vi "Write Time Measurement Requested 2.vi"(8 "error in (no error)":errorcluster, 10 "Time Measurement Requested":timestamp, 11 "Launch Measurements Message in":refnum<class "Launch Measurements Message.lvclass">) -> (0 "error out":errorcluster, 3 "Launch Measurements Message out":refnum<class "Launch Measurements Message.lvclass">)   [LabVIEW 2015, in "Controller Actor.lvlib" / "Launch Measurements Message.lvclass"]
uses:
  Launch Measurements Message.lvclass
  Launch Measurements Message.lvclass/Launch Measurements Message.ctl
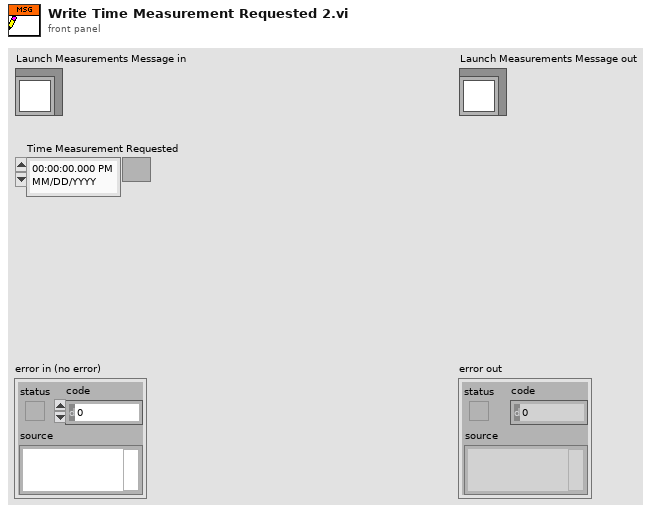
[diagram p1: front panel]
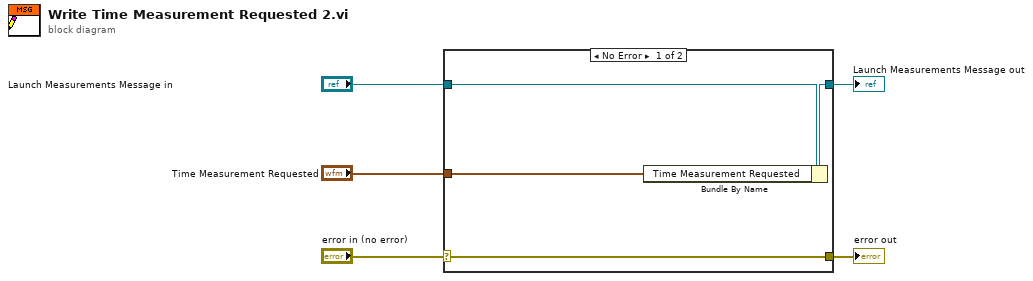
[diagram p0: block diagram]
diagram:
  n1 = case shown="No Error" "error in (no error)" {
    selector: "error in (no error)" -> [w9 w10]
    tunnel: [w9 w10] -> w4
    tunnel: [w7 w11] -> w2
    tunnel: "Launch Measurements Message in" -> [w8 w11]
    tunnel: "Time Measurement Requested" -> [w6 _]
    frame No Error {
      n2 = Bundle By Name(cluster=w8, "Time Measurement Requested"=w6) -> (w7:refnum<class "Launch Measurements Message.lvclass">)
    }
    frame Error {
    }
  }
  "error out" <- w4
  "Launch Measurements Message out" <- w2
